vi "Metronome Launch.vi"   [LabVIEW 2011, in "Messenging.lvlib" / "Metronome.lvclass"]
uses:
  Metronome.lvclass
  Interprocess Messenger/Send/Send.lvclass
  Interprocess Messenger/Send/Send Variant.vi
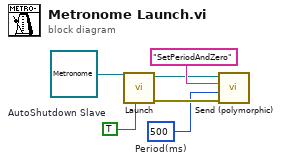
[diagram p0: block diagram]
diagram:
  w1 = TRUE  # AutoShutdown Slave
  w2 = 500  # Period(ms)
  n1 = call-dynamic "Launch.vi"("AutoShutdown Slave (F)"=w1, "Parallel Process in"=refnum<class "Metronome.lvclass"> refnum ("Metronome")) -> ("error out"=w3:errorcluster, "Parallel Process out"=w4:refnum<class "Metronome.lvclass">)  [unwired: 2 in, 6 out]
  n2 = call-poly "Send (polymorphic).vi"("error in (no error)"=w3, "Varient"=w2, "Label"="SetPeriodAndZero", "MSR Parent in"=w4) -> ()  [unwired: 8 out]
